vi "TestReadFromMote.vi"() -> ()   [LabVIEW 2010]
uses:
  <vilib>/picture/picture.llb/Draw True-Color Pixmap.vi
panel:
  out "bytes read":i32
  out "Counter":i16(graph)
  out "Dummy":sgl
  in  "header size":i32
  in  "bytes to read":i32
  out "Packet Payload":string
  in  "Enable Read":bool=TRUE
  in  "Port Number":i32=9002
  out "KTH  Automatic Control \nTemplates. Read from SerialForwarder":picture
  # "For TestSerialCommMsg:\nheaderSize = 9\npayload = 4"
  # "Communication control"
  # "Communication results"
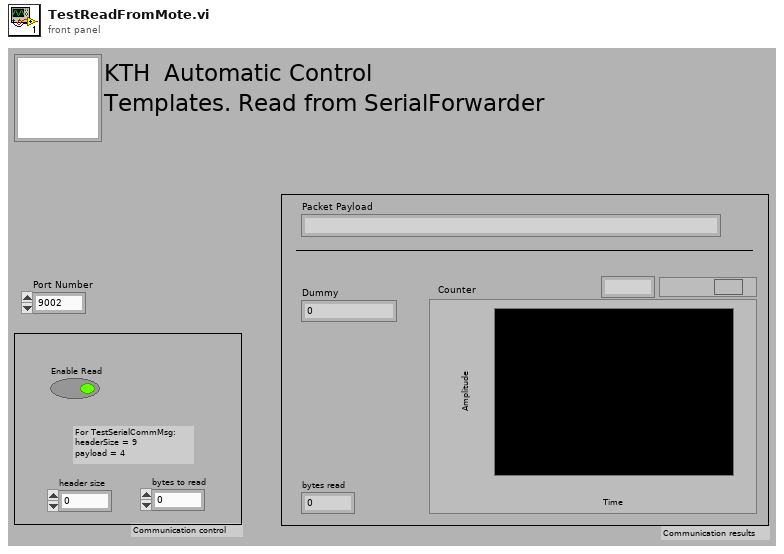
[diagram p1: front panel]
types:
  T1 = typedef "imagedata.ctl" = cluster{"image type":i32, "image depth":i32, "image":u8[], "mask":u8[], "colors":u32[], "Rectangle":cluster{"left":i16, "top":i16, "right":i16, "bottom":i16}}
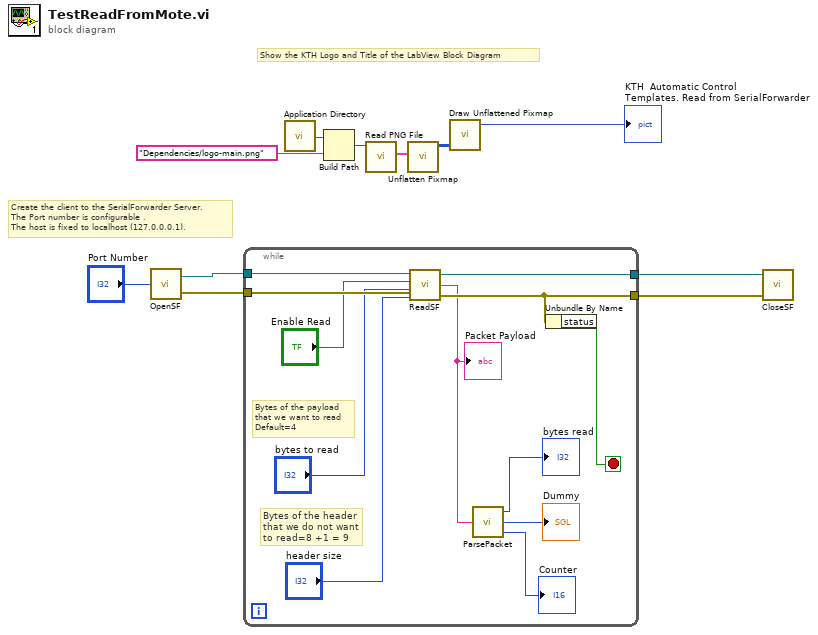
[diagram p0: block diagram]
diagram:
  # "Create the client to the SerialForwarder Server.\nThe Port number is configurable . \nThe host is fixed to localhost (127.0.0.0.1)."
  # "Show the KTH Logo and Title of the LabView Block Diagram"
  n1 = call "OpenSF.vi"("Port Number"="Port Number") -> ("error out"=w10:errorcluster, "connection ID"=w11:refnum<k5>)
  n2 = while {
    tunnel: w11 -> [w22]
    tunnel: w10 -> [w23]
    tunnel: [w21] -> w9
    tunnel: [w19] -> w8
    stop <- w20 stop-if-true
    # "Bytes of the payload \nthat we want to read\nDefault=4"
    # "Bytes of the header\nthat we do not want \nto read=8 +1 = 9"
    n3 = call "ReadSF.vi"("connection ID in"=w22, "enabled"="Enable Read", "bytes to read"="bytes to read", "header size"="header size", "error in"=w23) -> ("connection ID out"=w21:refnum<k5>, "string"=w15:string, "error out"=w19:errorcluster)
    "Packet Payload" <- w15
    n4 = call "ParsePacket.vi"("data out"=w15) -> ("Counter"=→"Counter":i16, "Dummy"=→"Dummy":i16, "Bytes read"=→"bytes read":i32)
    n5 = Unbundle By Name(w19) -> ("status"=w20:bool)
  }
  n6 = call <vilib>:"Application Directory.vi"() -> ("Application Directory"=w3:path)
  n7 = Build Path(base path=w3, name or relative path="Dependencies/logo-main.png") -> (appended path=w4:path)
  n8 = call <vilib>:"Read PNG File.vi"("path to PNG file"=w4) -> ("image data"=w7:T1)  [unwired: 8 in, 2 out]
  n9 = call <vilib>:"Unflatten Pixmap.vi"("image data"=w7) -> ("24-bit pixmap"=w6:u32[][])  [unwired: 4 in, 6 out]
  n10 = call-poly <vilib>:"Draw Unflattened Pixmap.vi"("data (RGB format)"=w6) -> ("new picture"=→"KTH  Automatic Control \nTemplates. Read from SerialForwarder":picture)  [unwired: 8 in]
  n11 = call "CloseSF.vi"("error out"=w8, "connection ID"=w9) -> ()  [unwired: 1 in]
